vi "Falling Edge Detector.vi"() -> ()   [LabVIEW 2018]
panel:
  out "Falling edge?":bool
  in  "Input":bool
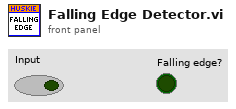
[diagram p1: front panel]
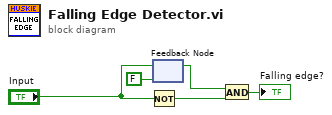
[diagram p0: block diagram]
diagram:
  n1 = Not(x="Input") -> (.not. x?=w1:bool)
  n2 = feedback #1(FALSE ("Input")) -> (w4:bool)
  n3 = feedback-in #1("Input") -> ()
  n4 = And(x=w4, y=w1) -> (x .and. y?=→"Falling edge?":bool)
